vi "globalTearDown.vi"(8 "error in (no error)":errorcluster, 11 "testcase-CSMSyncMessage in":refnum<class "testcase-CSMMessage.lvclass">) -> (0 "error out":errorcluster, 3 "testcase-CSMSyncMessage out":refnum<class "testcase-CSMMessage.lvclass">)   [LabVIEW 2017, in "testcase-CSMMessage.lvclass"]
uses:
  testcase-CSMMessage.lvclass
  testcase-CSMMessage.lvclass/testcase-CSMMessage.ctl
  <vilib>/addons/_JKI Toolkits/VI Tester/TestCase.llb/TestCase.lvclass
  src/user.lib/_NEVSTOP/Communicable State Machine(CSM)/_Support/Typedef/_CSM_List Module Scope.ctl
  src/user.lib/_NEVSTOP/Communicable State Machine(CSM)/Communicable State Machine.lvlib
panel:
  out "Module Names":string[](array[string])
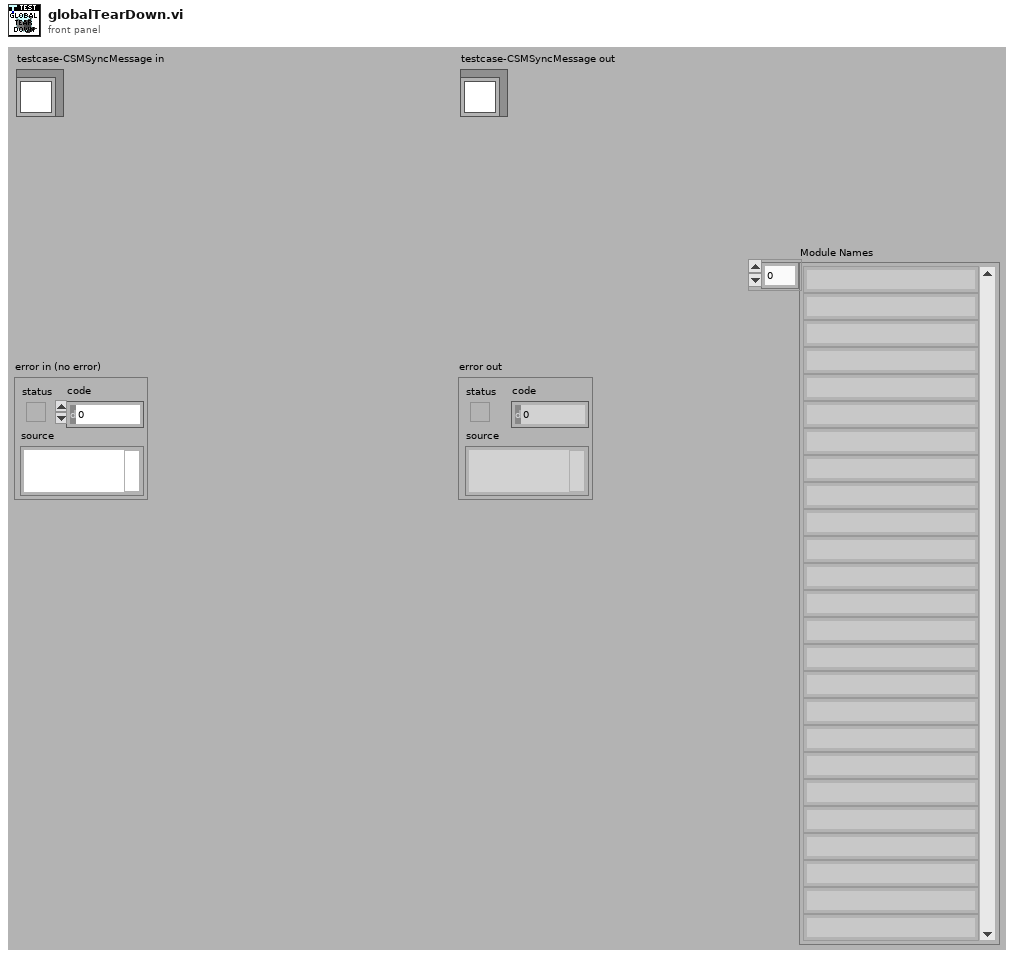
[diagram p1: front panel]
types:
  T1 = typedef "Communicable State Machine.lvlib/_CSM_List Module Scope.ctl" = enum16{"Normal", "System Only", "All"}
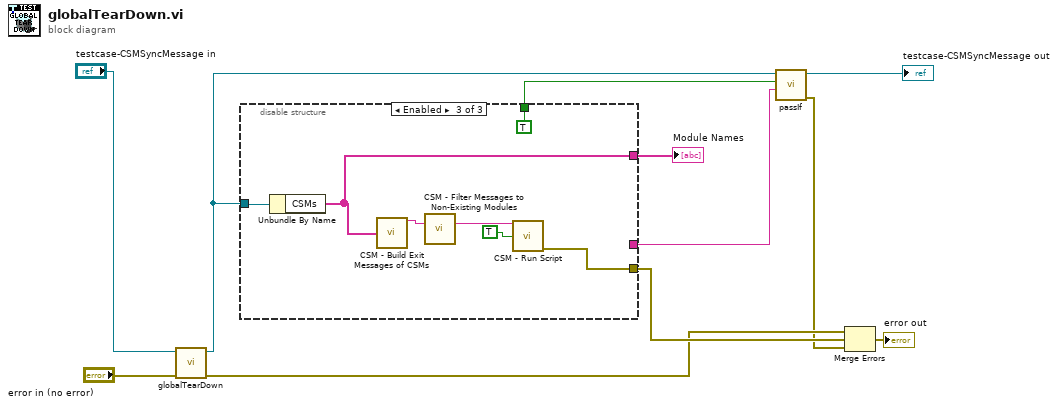
[diagram p0: block diagram]
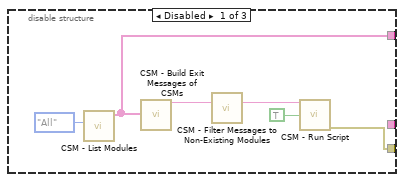
[diagram p2: hidden frame]
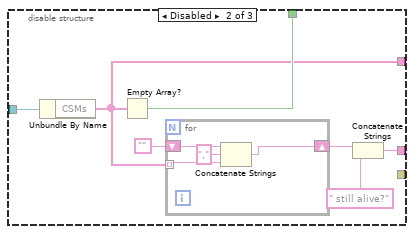
[diagram p3: hidden frame]
diagram:
  n1 = call-parent "globalTearDown.vi"("error in (no error)"="error in (no error)", "TestCase in"="testcase-CSMSyncMessage in") -> ("error out"=w2:errorcluster, "TestCase out"=w4:refnum<class "testcase-CSMMessage.lvclass">)  [unwired: 8 in]
  n2 = disable-structure shown="Enabled" {
    disable-tunnel: [w13 _ w30] -> w6
    disable-tunnel: w4 -> [_ w24 w35]
    disable-tunnel: [w12 w22 w31] -> w9
    disable-tunnel: [_ w23 TRUE ("pass")] -> w8
    disable-tunnel: [_ w18 _] -> w7
    frame Disabled {
      n3 = call "CSM - List Modules.vi"("Scope (Normal)"=_CSM_List_Module_Scope."All") -> ("Module Names"=w12:string[])  [unwired: 9 in, 1 out]
      n4 = call "CSM - Build Exit Messages of CSMs.vi"("CSMs"=w12) -> ("States"=w17:string)  [unwired: 14 in]
      n5 = call "CSM - Filter Messages to Non-Existing Modules.vi"("States In"=w17) -> ("States Out"=w15:string)  [unwired: 14 in]
      n6 = call "CSM - Run Script.vi"("CSM Scripts"=w15, "Continue If Error? (F)"=TRUE) -> ("error out"=w13:errorcluster)  [unwired: 11 in, 2 out]
    }
    frame Disabled {
      n7 = Unbundle By Name(w24) -> ("CSMs"=w22:string[])
      n8 = Empty Array?(array=w22) -> (empty?=w23:bool)
      n9 = for {
        tunnel: w22 -> [w26] mode=indexing
        shift-right: [w27] -> w20
        shift-left: "" -> [w28]
        n10 = Concatenate Strings(w28, "," ("string"), w26) -> (w27:string)
      }
      n11 = Concatenate Strings(w20, " still alive?" ("string")) -> (w18:string)
    }
    frame Enabled {
      n12 = Unbundle By Name(w35) -> ("CSMs"=w31:string[])
      n13 = call "CSM - Build Exit Messages of CSMs.vi"("CSMs"=w31) -> ("States"=w34:string)  [unwired: 14 in]
      n14 = call "CSM - Filter Messages to Non-Existing Modules.vi"("States In"=w34) -> ("States Out"=w32:string)  [unwired: 14 in]
      n15 = call "CSM - Run Script.vi"("CSM Scripts"=w32, "Continue If Error? (F)"=TRUE) -> ("error out"=w30:errorcluster)  [unwired: 11 in, 2 out]
    }
  }
  "Module Names" <- w9
  n16 = call-dynamic "passIf.vi"("message (\"\")"=w7, "pass"=w8, "TestCase in"=w4) -> ("error out"=w1:errorcluster, "TestCase out"=→"testcase-CSMSyncMessage out":refnum<class "testcase-CSMMessage.lvclass">)  [unwired: 7 in]
  n17 = Merge Errors(w2, w6, w1) -> (→"error out":errorcluster)
